vi "Stop Heat.vi"(8 "error in (no error)":errorcluster, 11 "Oven Actor in":refnum<class "Oven Actor.lvclass">) -> (0 "error out":errorcluster, 3 "Oven Actor out":refnum<class "Oven Actor.lvclass">)   [LabVIEW 2021, in "Oven Actor.lvlib" / "Oven Actor.lvclass"]
uses:
  Oven Actor.lvclass
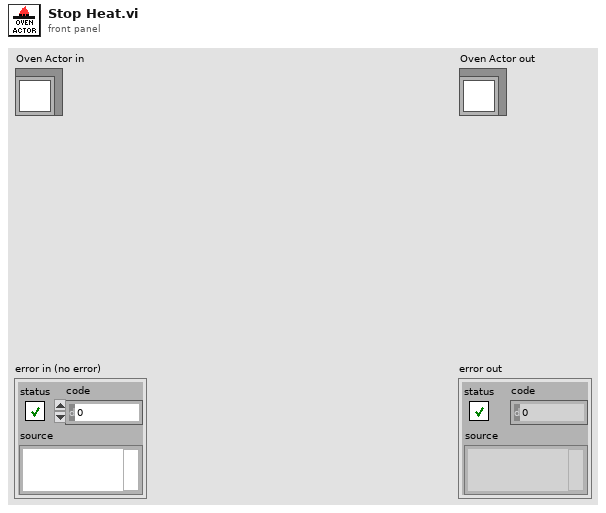
[diagram p1: front panel]
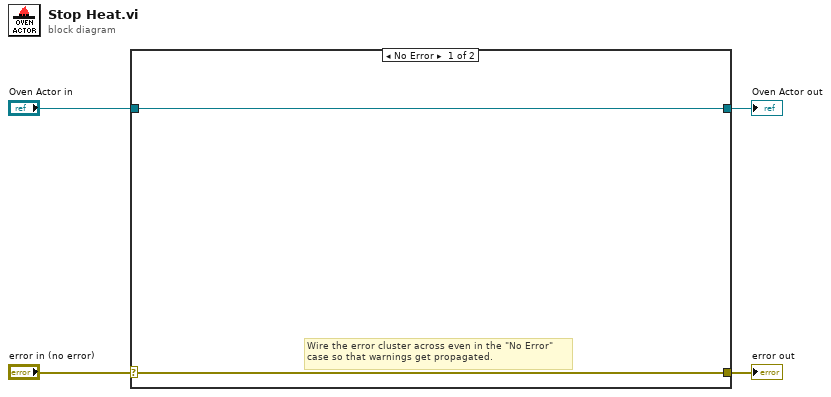
[diagram p0: block diagram]
diagram:
  n1 = case shown="No Error" "error in (no error)" {
    selector: "error in (no error)" -> [w5 w8]
    tunnel: [w5 w8] -> w3
    tunnel: [w6 w7] -> w1
    tunnel: "Oven Actor in" -> [w6 w7]
    frame No Error {
      # "Wire the error cluster across even in the \"No Error\"\ncase so that warnings get propagated."
    }
    frame Error {
    }
  }
  "error out" <- w3
  "Oven Actor out" <- w1
